vi "Update Log_OccupancyGrid Cell cost.vi"(6 "cell cost":dbl, 8 "error in (no error)":errorcluster, 9 "Y_map":i32, 10 "X_map":i32, 11 "Probabilistic_OccupancyGrid in":refnum<class "Probabilistic_OccupancyGrid.lvclass">) -> (0 "error out":errorcluster, 3 "Probabilistic_OccupancyGrid out":refnum<class "Probabilistic_OccupancyGrid.lvclass">)   [LabVIEW 2017, in "Probabilistic_OccupancyGrid.lvclass"]
uses:
  Probabilistic_OccupancyGrid.lvclass
  Probabilistic_OccupancyGrid.lvclass/Probabilistic_OccupancyGrid.ctl
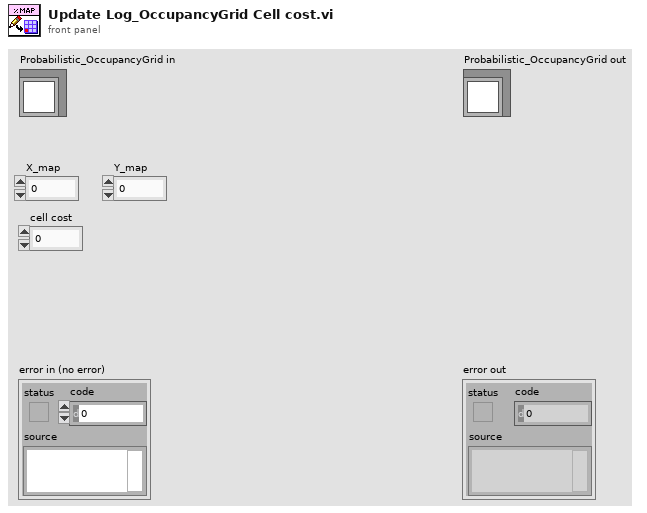
[diagram p1: front panel]
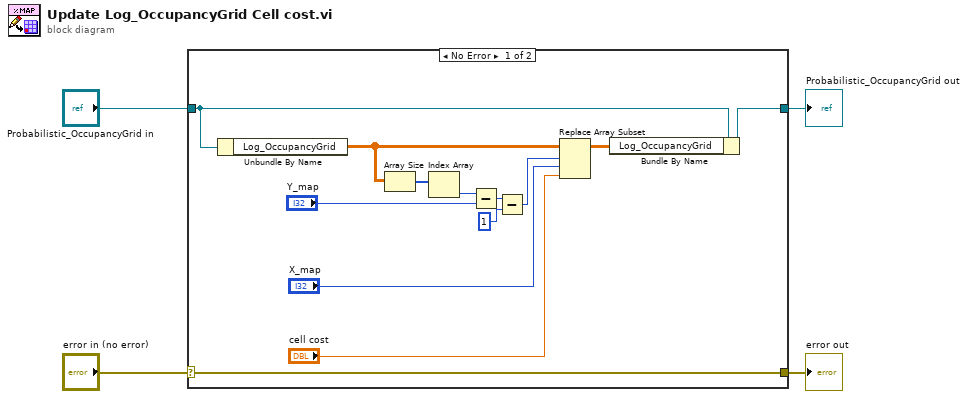
[diagram p0: block diagram]
diagram:
  n1 = case shown="No Error" "error in (no error)" {
    selector: "error in (no error)" -> [w17 w19]
    tunnel: [w17 w19] -> w3
    tunnel: [w5 w18] -> w1
    tunnel: "Probabilistic_OccupancyGrid in" -> [w7 w18]
    frame No Error {
      n2 = Unbundle By Name(w7) -> ("Log_OccupancyGrid"=w8:dbl[][])
      n3 = Array Size(array=w8) -> (size(s)=w13:i32[])
      n4 = Index Array(array=w13) -> (element=w14:i32)  [unwired: 1 in]
      n5 = Subtract(x=w14, y="Y_map") -> (x-y=w11:i32)
      n6 = Subtract(x=w11, y=1) -> (x-y=w9:i32)
      n7 = Replace Array Subset(array=w8, new element="cell cost", index (row)=w9, index (col)="X_map") -> (w6:dbl[][])
      n8 = Bundle By Name(cluster=w7, "Log_OccupancyGrid"=w6) -> (w5:refnum<class "Probabilistic_OccupancyGrid.lvclass">)
    }
    frame Error {
    }
  }
  "error out" <- w3
  "Probabilistic_OccupancyGrid out" <- w1
